vi "K calc.vi"(1 "Current Head":dbl format="%.2f", 2 "Initial Head":dbl format="%.2f", 3 "Flow":dbl format="%.2f") -> (0 "K":dbl format="%.2f")   [LabVIEW 2016]
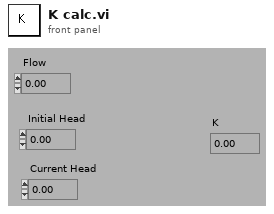
[diagram p1: front panel]
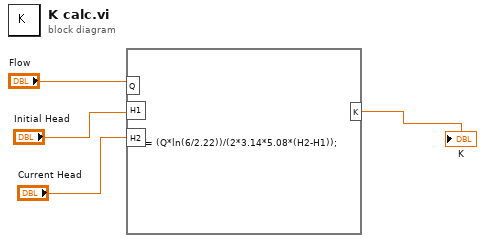
[diagram p0: block diagram]
diagram:
  n1 = formula code="K = (Q*ln(6/2.22))/(2*3.14*5.08*(H2-H1));"("Q"="Flow", "H1"="Initial Head", "H2"="Current Head") -> ("K"=→"K":dbl)
